vi "String Array to Comma Separated Strings.vi"(1 "String Array":string[](array[string])) -> (15 "Comma Separated Strings":string)   [LabVIEW 2015, in "RT Management.lvlib" / "Module Detection.lvclass"]
uses:
  Module Detection.lvclass
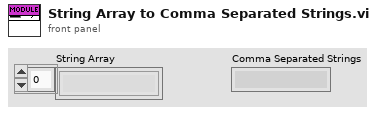
[diagram p1: front panel]
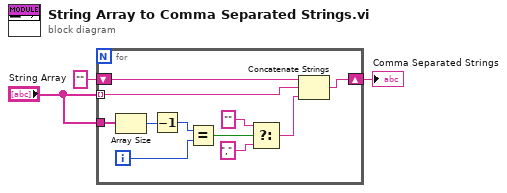
[diagram p0: block diagram]
diagram:
  n1 = for {
    tunnel: "String Array" -> [w14] mode=indexing
    tunnel: "String Array" -> [w11]
    shift-right: [w13] -> w1
    shift-left: "" -> [w12]
    i -> [w8]
    n2 = Array Size(array=w11) -> (size(s)=w10:i32)
    n3 = Decrement(x=w10) -> (x-1=w9:i32)
    n4 = Equal?(x=w9, y=w8) -> (x = y?=w7:bool)
    n5 = Select(t="", s=w7, f="," ("string")) -> (s? t:f=w5:string)
    n6 = Concatenate Strings(w12, w14, w5) -> (w13:string)
  }
  "Comma Separated Strings" <- w1
